vi "Do.vi"(8 "error in (no error)":errorcluster, 10 "Actor in":refnum<class "Actor.lvclass">, 11 "Init Msg":refnum<class "Init Msg.lvclass">) -> (0 "error out":errorcluster, 2 "Actor out":refnum<class "Actor.lvclass">)   [LabVIEW 2020, in "CameraTestingProxy.lvlib" / "Init Msg.lvclass"]
doc: "This VI delivers the message to the actor by calling the appropriate method(s) on the actor."
uses:
  Init Msg.lvclass
  <vilib>/ActorFramework/Actor/Actor.lvclass
  CameraTestingENI/CameraTestingENI.lvclass
  C:/Program Files (x86)/National Instruments/LabVIEW 2020/vi.lib/ActorFramework/Actor/Actor.lvclass
  9ef47adc-f318-494c-9b8b-6df3216d6863.vi
  Init Msg.lvclass/Init Msg.ctl
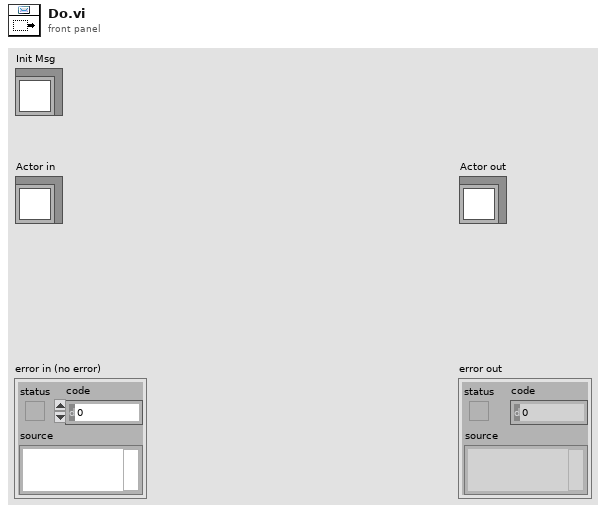
[diagram p1: front panel]
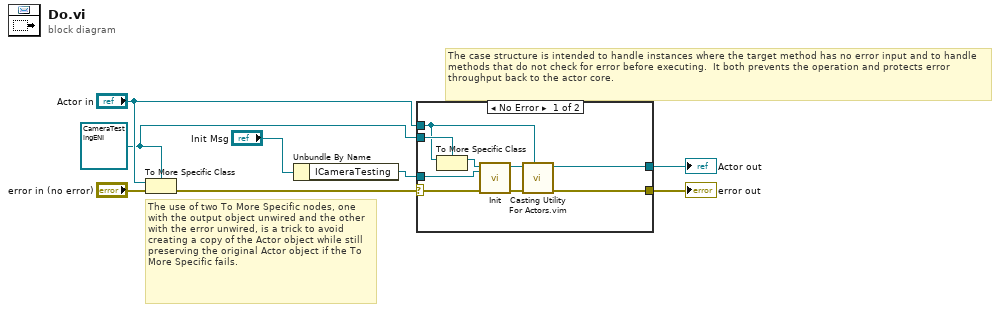
[diagram p0: block diagram]
diagram:
  w3 = refnum<class "CameraTestingENI.lvclass"> refnum ("Actor in")
  # "The use of two To More Specific nodes, one with the output object unwired and the other with the error unwired, is a trick to avoid creating a copy of the Actor object while still preserving the original Actor object if the To More Specific fails."
  # "The case structure is intended to handle instances where the target method has no error input and to handle methods that do not check for error before executing.  It both prevents the operation and protects error throughput back to the actor core."
  n1 = To More Specific Class(target class=w3, reference="Actor in", error in="error in (no error)") -> (error out=w7:errorcluster)  [unwired: 1 out]
  n2 = Unbundle By Name("Init Msg") -> ("ICameraTesting"=w1:refnum<class "ICameraTesting.lvclass">)
  n3 = case shown="No Error" w7 {
    selector: w7 -> [w17 w19]
    tunnel: [w11 w19] -> w6
    tunnel: [w12 w18] -> w5
    tunnel: "Actor in" -> [w14 w18]
    tunnel: w3 -> [w15 _]
    tunnel: w1 -> [w9 _]
    frame No Error {
      n4 = To More Specific Class(target class=w15, reference=w14) -> (specific class reference=w16:refnum<class "CameraTestingENI.lvclass">)  [unwired: 1 in, 1 out]
      n5 = call "Init.vi"("error in (no error)"=w17, "ICameraTesting"=w9, "CameraTestingUI in"=w16) -> ("error out"=w10:errorcluster, "CameraTestingUI out"=w13:refnum<class "CameraTestingENI.lvclass">)  [unwired: 7 in]
      n6 = call "Casting Utility For Actors.vim"("type"=w14, "error in (no error)"=w10, "Actor in"=w13) -> ("error out"=w11:errorcluster, "Actor out"=w12:refnum<class "Actor.lvclass">)  [unwired: 7 in]
    }
    frame Error {
      # "If type check fails, pass the original object out again."
    }
  }
  "error out" <- w6
  "Actor out" <- w5
